vi "QTrkBeginLUT.vi"(4 "error in (no error)":errorcluster, 6 "Normalize (T)":bool=TRUE, 7 "QTrk Instance":T1) -> (0 "error out":errorcluster, 3 "QTrk Instance":T1)   [LabVIEW 2011]
uses:
  QTrkInstance.ctl
  QTrkDLL.vi
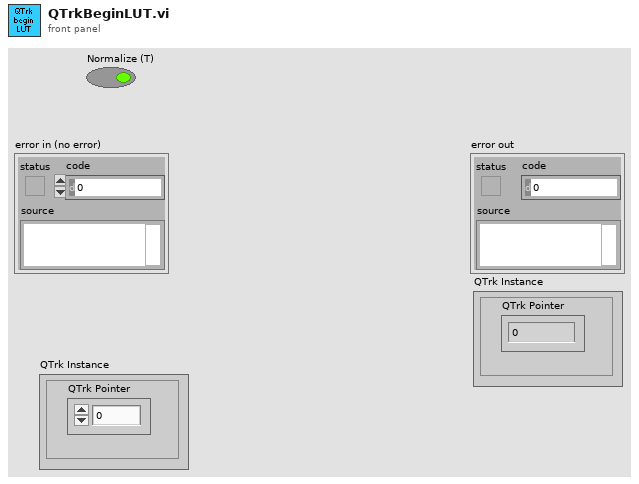
[diagram p1: front panel]
types:
  T1 = typedef "QTrkInstance.ctl" = cluster{"QTrk Pointer":u64}
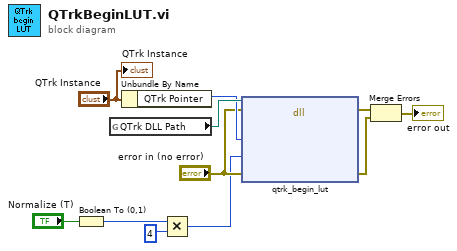
[diagram p0: block diagram]
diagram:
  n1 = Boolean To (0,1)(Boolean="Normalize (T)") -> (0, 1=w3:i16)
  n2 = global read "QTrkDLL.vi" "QTrk DLL Path"() -> (w11:path)
  n3 = Unbundle By Name("QTrk Instance") -> ("QTrk Pointer"=w9:u64)
  n4 = Multiply(x=w3, y=i16 4) -> (x*y=w1:i16)
  n5 = dll-call lib="D:/jcnossen1/cudaqi-tracker/cudatrack-labview/cputrack_d.dll" fn="qtrk_begin_lut"(path in=w11, error in="error in (no error)", "tracker"=w9, "flags"=w1, "error"="error in (no error)") -> (error out=w7:errorcluster, "error"=w6:errorcluster)  [unwired: 4 in, 1 out]
  n6 = Merge Errors(w7, w6) -> (→"error out":errorcluster)
  "QTrk Instance" <- "QTrk Instance"
